vi "fgt set power.vi"(8 "error in (no error)":errorcluster, 10 "powerState":T1, 11 "controllerIndex":u16) -> (0 "error out":errorcluster)   [LabVIEW 2016, in "fgt_SDK.lvlib"]
doc: "Set power ON or OFF on a controller (such as Link, MFCS, Flowboard).\nNot all controllers support this functionality."
uses:
  fgt_SDK.lvlib
  TypeDefs/fgt_POWER.ctl
  dlls/fgt_SDK_32.dll
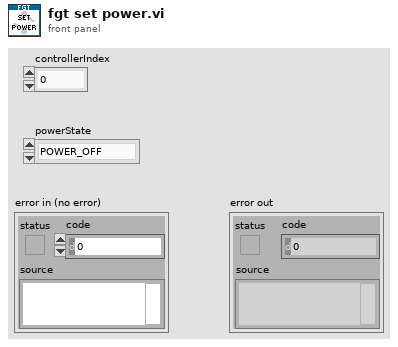
[diagram p1: front panel]
types:
  T1 = typedef "fgt_SDK.lvlib/fgt_POWER.ctl" = enum8{"POWER_OFF", "POWER_ON", "SLEEP"}
  T2 = typedef "fgt_SDK.lvlib/fgt_STATUS_INFO.ctl" = cluster{"InstrType":T3, "instrSN":u16, "errorCode":u8, "infoCode":u8, "detail":string}
  T3 = typedef "fgt_SDK.lvlib/fgt_INSTRUMENT_TYPE.ctl" = enum32{"None", "MFCS", "MFCS_EZ", "FRP", "LineUP"}
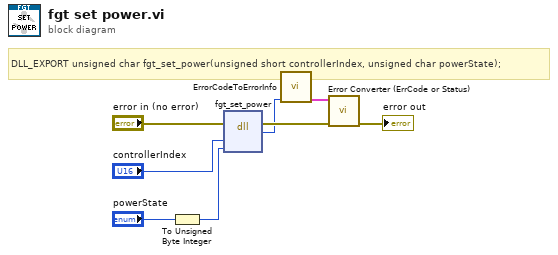
[diagram p0: block diagram]
diagram:
  # "DLL_EXPORT unsigned char fgt_set_power(unsigned short controllerIndex, unsigned char powerState);"
  n1 = To Unsigned Byte Integer(number="powerState") -> (unsigned 8bit integer=w3:u8)
  n2 = dll-call lib="PTH2Zabs D\nMes DocumentsDéveloppementFluigentSDKsfgt-sdk-labviewdllsfgt_SDK_*.*" fn="fgt_set_power"(error in="error in (no error)", "controllerIndex"="controllerIndex", "powerState"=w3) -> (error out=w6:errorcluster, "return type"=w2:u8)  [unwired: 4 in, 1 out]
  n3 = call "ErrorCodeToErrorInfo.vi"("return type"=w2) -> ("StatusInfo"=w1:T2)  [unwired: 10 in]
  n4 = call "Error Converter (ErrCode or Status).vi"("error in (no error)"=w6, "StatusInfo"=w1) -> ("error out"=→"error out":errorcluster)  [unwired: 9 in]
